vi "SDO upload.vi"(4 "Size":u8=4, 5 "Destination":refnum<vi>, 6 "error in (no error)":errorcluster, 7 "Multiplexor":T1 {"Sub-Index" format="%.0x"; "Index" format="%04x"}, 8 "Node ID":u16, 9 "CANopen in":refnum<class "CANopen.lvclass">) -> (0 "error out":errorcluster, 3 "CANopen out":refnum<class "CANopen.lvclass">)   [LabVIEW 2026, in "canopen_.lvlib" / "CANopen.lvclass"]
doc: "Reads an entry from the open dictionary of a CANopen node."
uses:
  CANopen.lvclass
  CANopen.lvclass/CANopen.ctl
  FunctionCode.ctl
  CANopen Master.lvlib
  Multiplexor.ctl
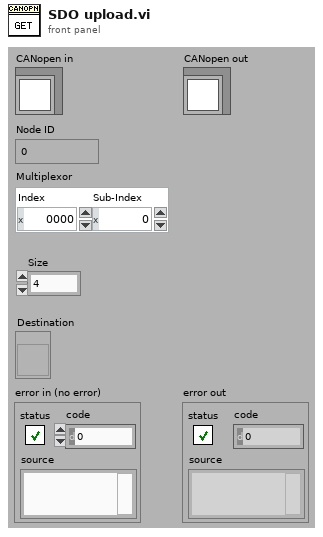
[diagram p1: front panel]
types:
  T1 = typedef "CANopen Master.lvlib/Multiplexor.ctl" = cluster{"Index":u16, "Sub-Index":i16}
  T2 = typedef "CANopen Master.lvlib/FunctionCode.ctl" = u16
  T3 = cluster{"COD-ID":u32, u8, "Size":u8, "Destination":refnum<vi>}
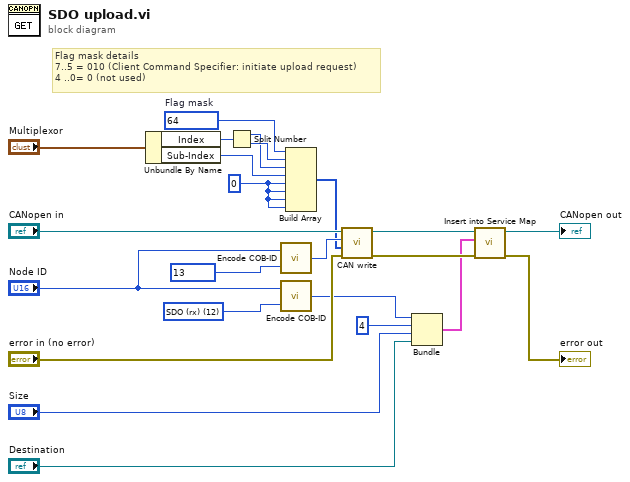
[diagram p0: block diagram]
diagram:
  w14 = T2 12 items=["EMCY"=1, "PDO1 (tx)"=3, "PDO1 (rx)"=4, "PDO2 (tx)"=5, "PDO2 (rx)"=6, "PDO3 (tx)"=7, "PDO3 (rx)"=8, "PDO4 (tx)"=9, "PDO4 (rx)"=10, "SDO (tx)"=11, "SDO (rx)"=12, "NMT error control"=14] ("Function code")
  w16 = u8 0 ("element")
  w8 = T2 13 items=["EMCY"=1, "PDO1 (tx)"=3, "PDO1 (rx)"=4, "PDO2 (tx)"=5, "PDO2 (rx)"=6, "PDO3 (tx)"=7, "PDO3 (rx)"=8, "PDO4 (tx)"=9, "PDO4 (rx)"=10, "SDO (tx)"=11, "SDO (rx)"=12, "NMT error control"=14] ("Function code")
  w17 = u8 64  # Flag mask
  # "Flag mask details\n7..5 = 010 (Client Command Specifier: initiate upload request)\n4 ..0= 0 (not used)"
  n1 = Unbundle By Name("Multiplexor") -> ("Index"=w21:u16, "Sub-Index"=w18:i16)
  n2 = Split Number(x=w21) -> (hi(x)=w19:u8, lo(x)=w20:u8)
  n3 = call "Encode COB-ID.vi"("Function code"=w8, "Node-ID"="Node ID") -> ("COD-ID"=w7:u32)
  n4 = call "Encode COB-ID.vi"("Function code"=w14, "Node-ID"="Node ID") -> ("COD-ID"=w13:u32)
  n5 = Build Array(w17, w20, w19, w18, w16, w16, w16, w16) -> (w5:i16[])
  n6 = call "CAN write.vi"("error in (no error)"="error in (no error)", "Data"=w5, "COB id"=w7, "CANopen in"="CANopen in") -> ("error out"=w10:errorcluster, "CANopen out"=w12:refnum<class "CANopen.lvclass">)  [unwired: 2 out]
  n7 = Bundle("COD-ID"=w13, u8 4, "Size"="Size", "Destination"="Destination") -> (w2:T3)  [unwired: 1 out]
  n8 = call "Insert into Service Map.vi"("error in"=w10, 6:w2, "CANopen in"=w12) -> ("error out"=→"error out":errorcluster, "CANopen out"=→"CANopen out":refnum<class "CANopen.lvclass">)  [unwired: 3 out]
